vi "simple test API.vi"() -> ()   [LabVIEW 2013]
uses:
  dynamic profibus/full response.ctl
  dynamic profibus/profibus master transmit header.ctl
  dynamic profibus/full command.ctl
  dynamic profibus/profibus master action.ctl
  <vilib>/FPGAPlugInAG/cRIO-9068/niLvFpga_Open_cRIO-9068.vi
  <vilib>/rvi/interface/common/dynamic/niFpgaDynamicAddResources.vi
  <vilib>/FPGAPlugInAG/Dynamic/niLvFpga_Reset_Dynamic.vi
  <vilib>/FPGAPlugInAG/Dynamic/niLvFpga_Run_Dynamic.vi
  <vilib>/FPGAPlugInAG/Dynamic/niLvFpga_Close_Dynamic.vi
  <vilib>/rvi/interface/nirviOpenFPGA/nirviOpenFPGA.xnode
  FPGA Bitfiles/ProfibusModule_FPGATargetMSlave_FPGAMain_hsONVj+8C84.lvbitx
  execution/FPGA Main.vi
  <vilib>/rvi/interface/nirviMethod/nirviMethod.xnode
  <vilib>/rvi/interface/nirviCloseFPGA/nirviCloseFPGA.xnode
  dynamic profibus/dynamic profibus.lvlib
panel:
  out "responses":T1[](array[typedef])
  out "Slave Info List":T3(array[cluster])
  out "error out":errorcluster
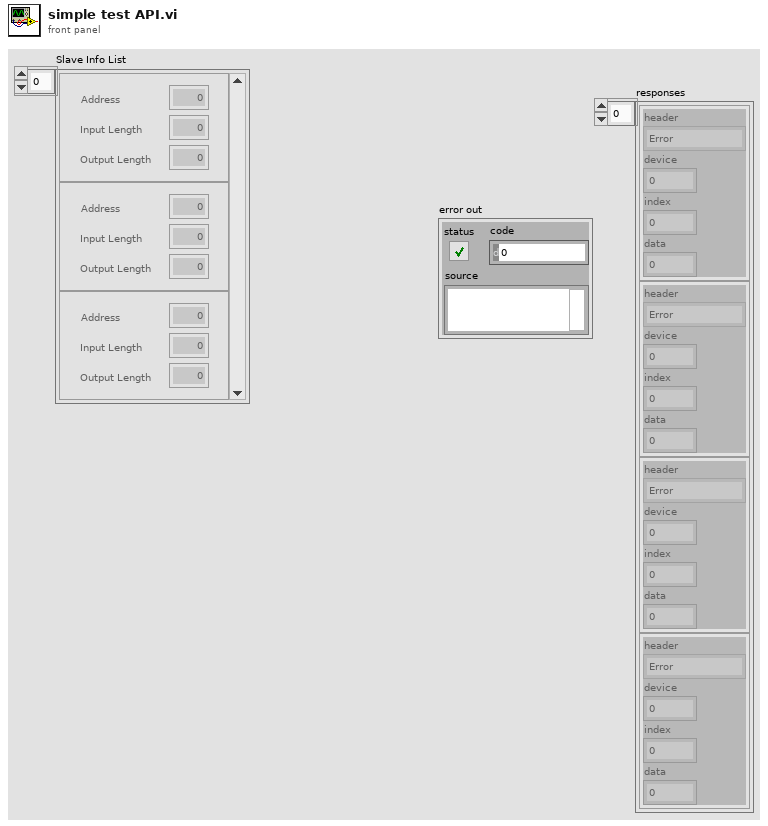
[diagram p1: front panel]
types:
  T1 = typedef "dynamic profibus.lvlib/full response.ctl" = cluster{"header":T2, "device":u8, "index":u8, "data":u8}
  T2 = typedef "dynamic profibus.lvlib/profibus master transmit header.ctl" = enum8{"Error", "Input", "Diagnostic", "input size", "output size"}
  T3 = cluster{"Address":i8, "Input Length":u8, "Output Length":u8}[]
  T4 = typedef "dynamic profibus.lvlib/full command.ctl" = cluster{"action":T5, "device":u8, "index":u8, "data":u8}
  T5 = typedef "dynamic profibus.lvlib/profibus master action.ctl" = enum8{"initialize", "uninitialize", "stop", "get input", "get input size", "set output", "get output size", "get diagnostic", "transfer data", "transfer diagnostics"}
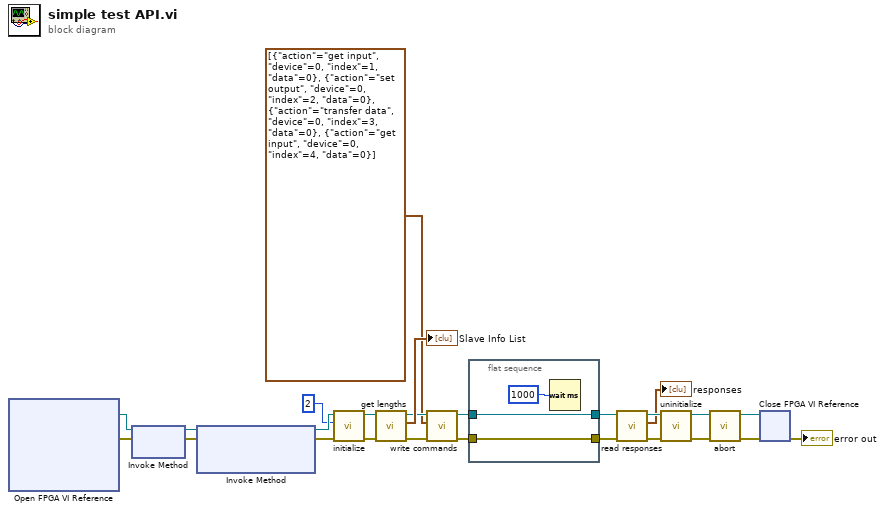
[diagram p0: block diagram]
diagram:
  n1 = xnode "Open FPGA VI Reference"() -> ("FPGA VI Reference Out"=w21:refnum<k20>, "error out"=w23:errorcluster)  [unwired: 2 in]
  n2 = xnode "Invoke Method"("FPGA VI Reference In"=w21, "error in"=w23) -> ("FPGA VI Reference Out"=w19:refnum<k20>, "error out"=w22:errorcluster)
  n3 = xnode "Invoke Method"("FPGA VI Reference In"=w19, "error in"=w22) -> ("FPGA VI Reference Out"=w18:refnum<k20>, "error out"=w20:errorcluster)  [unwired: 1 in]
  n4 = call "initialize.vi"("error in"=w20, "device (if slave)"=u8 2, "profibus reference"=w18) -> ("error out"=w25:errorcluster, "profibus reference out"=w24:refnum<k20>)  [unwired: 7 in]
  n5 = call "get lengths.vi"("error in"=w25, "profibus reference"=w24) -> ("error out"=w10:errorcluster, "Slave Info List"=→"Slave Info List":T3, "profibus reference out"=w11:refnum<k20>)  [unwired: 7 in]
  n6 = call "write commands.vi"("error in"=w10, "commands"=T4[] [{"action"=enum."get input", "device"=0, "index"=1, "data"=0}, {"action"=enum."set output", "device"=0, "index"=2, "data"=0}, {"action"=enum."transfer data", "device"=0, "index"=3, "data"=0}, {"action"=enum."get input", "device"=0, "index"=4, "data"=0}], "profibus reference"=w11) -> ("error out"=w4:errorcluster, "profibus reference out"=w7:refnum<k20>)  [unwired: 7 in]
  n7 = flat-sequence {
    tunnel: w7 -> [w27]
    tunnel: [w27] -> w6
    tunnel: [w26] -> w5
    tunnel: w4 -> [w26]
    frame #0 {
      n8 = Wait (ms)(milliseconds to wait=u32 1000) -> ()  [unwired: 1 out]
    }
  }
  n9 = call "read responses.vi"("error in"=w5, "profibus reference"=w6) -> ("error out"=w8:errorcluster, "responses"=→"responses":T1[], "profibus reference out"=w9:refnum<k20>)  [unwired: 7 in]
  n10 = call "uninitialize.vi"("error in"=w8, "profibus reference"=w9) -> ("error out"=w16:errorcluster, "profibus reference out"=w17:refnum<k20>)  [unwired: 8 in]
  n11 = call "abort.vi"("error in"=w16, "profibus reference"=w17) -> ("error out"=w14:errorcluster, "profibus reference out"=w15:refnum<k20>)  [unwired: 8 in]
  n12 = xnode "Close FPGA VI Reference"("FPGA VI Reference In"=w15, "error in"=w14) -> ("error out"=→"error out":errorcluster)
